vi "Ch2-Ex1.vi"() -> ()   [LabVIEW 2019]
panel:
  out "Timer Done":bool
  in  "Wait Time\n(Seconds)":dbl
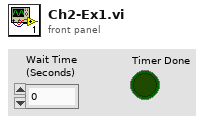
[diagram p1: front panel]
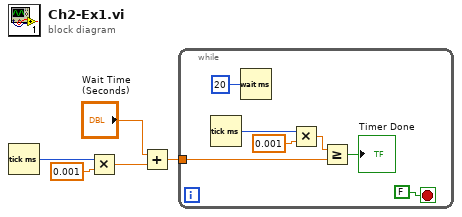
[diagram p0: block diagram]
diagram:
  n1 = Tick Count (ms)() -> (millisecond timer value=w5:u32)
  n2 = Multiply(x=w5, y=0.001) -> (x*y=w3:dbl)
  n3 = Add(x="Wait Time\n(Seconds)", y=w3) -> (x+y=w1:dbl)
  n4 = while {
    tunnel: w1 -> [w7]
    stop <- FALSE stop-if-true
    n5 = Tick Count (ms)() -> (millisecond timer value=w10:u32)
    n6 = Wait (ms)(milliseconds to wait=u32 20) -> ()  [unwired: 1 out]
    n7 = Multiply(x=w10, y=0.001) -> (x*y=w8:dbl)
    n8 = Greater Or Equal?(x=w8, y=w7) -> (x >= y?=→"Timer Done":bool)
  }
